vi "CreateSetTargetCommand.vi"(9 "Close communication":bool, 10 "Target value":i16, 11 "Sevo name":string) -> (3 "Command":u32[](array[numeric]))   [LabVIEW 2020]
doc: "Creates Set Target Command in Polulu Protocol as byte array."
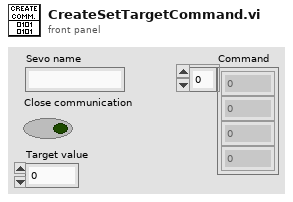
[diagram p1: front panel]
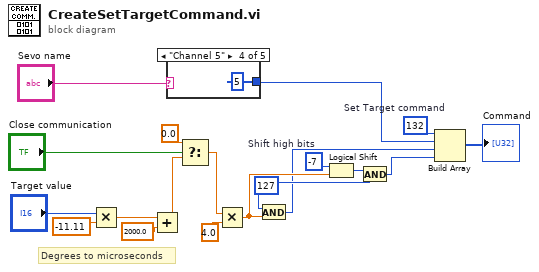
[diagram p0: block diagram]
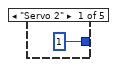
[diagram p2: hidden frame]
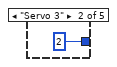
[diagram p3: hidden frame]
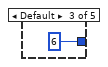
[diagram p4: hidden frame]
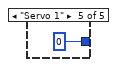
[diagram p5: hidden frame]
diagram:
  w14 = i8 -7  # Shift high bits
  w15 = u8 127
  w6 = u8 132  # Set Target command
  # "Degrees to microseconds"
  n1 = Multiply(x="Target value", y=-11.11) -> (x*y=w11:dbl)
  n2 = Add(x=w11, y=2000.0) -> (x+y=w3:dbl)
  n3 = case shown="\"Channel 5\"" "Sevo name" {
    tunnel: [u8 1 ("Servo") u8 2 ("Servo") u8 6 ("Servo") u8 5 ("Servo") u8 0 ("Servo")] -> w7
    frame "Servo 2" {
    }
    frame "Servo 3" {
    }
    frame Default {
    }
    frame "Channel 5" {
    }
    frame "Servo 1" {
    }
  }
  n4 = Select(t=0.0, s="Close communication", f=w3) -> (s? t:f=w2:dbl)
  n5 = Multiply(x=w2, y=4.0) -> (x*y=w16:dbl)
  n6 = And(x=w15, y=w16) -> (x .and. y?=w8:i32)
  n7 = Logical Shift(y=w14, x=w16) -> (x << y=w17:u32)
  n8 = And(x=w17, y=w15) -> (x .and. y?=w18:u32)
  n9 = Build Array(w6, w7, w8, w18) -> (→"Command":u32[])
